vi "STREAM_START.vi"(2 "error in (no error)":errorcluster, 3 "VISA resource Input":refnum<visa-resource-name>) -> (0 "error out":errorcluster, 1 "VISA resource name out":refnum<visa-resource-name>)   [LabVIEW 2011]
panel:
  out "Sent":u8[](array[numeric])
  out "return count":u32
  out "Read  Stream_Start command":u8[](array[numeric])
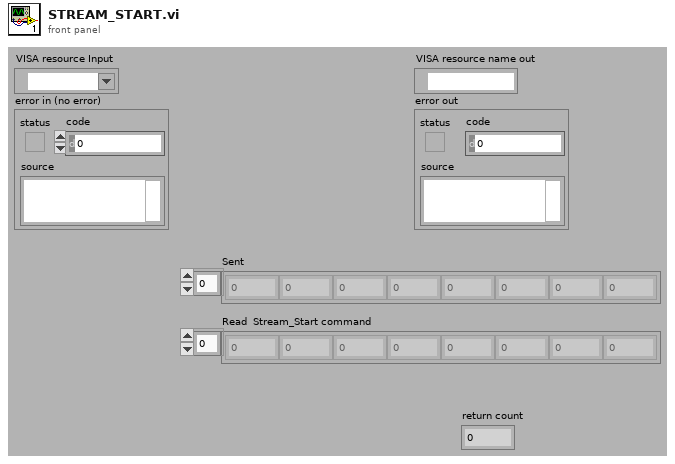
[diagram p1: front panel]
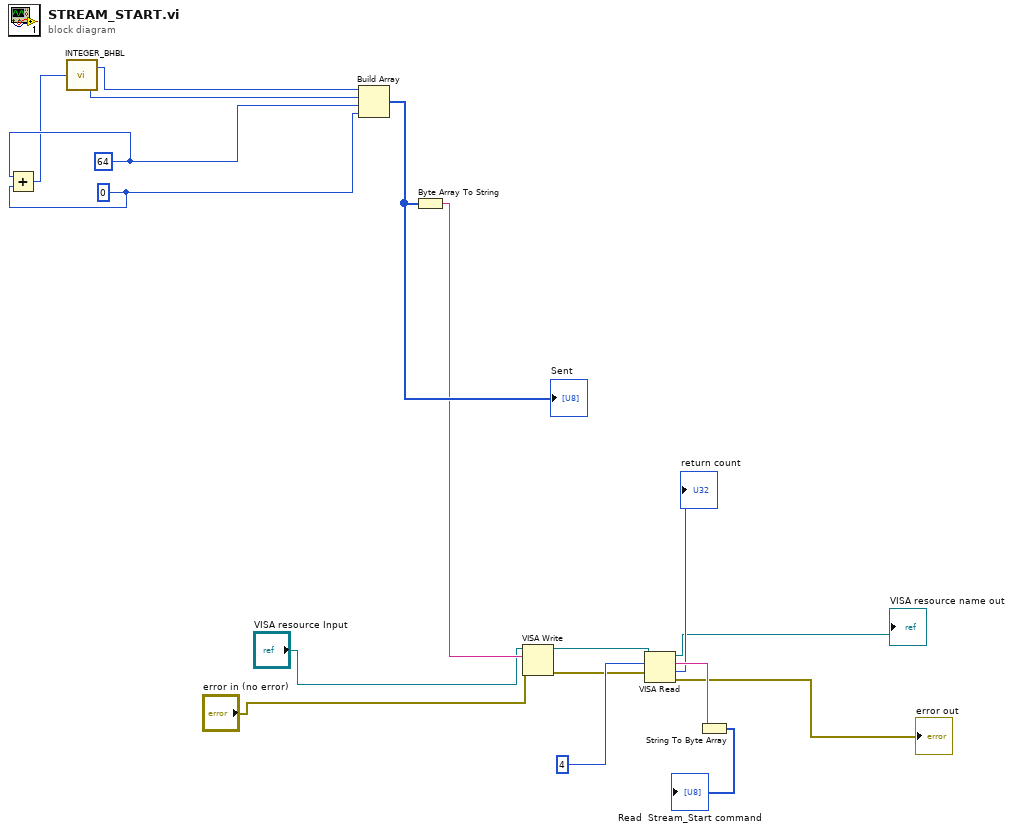
[diagram p0: block diagram]
diagram:
  w5 = i8 0 ("element")
  w4 = i8 64 ("element")
  n1 = Add(x=w4, y=w5) -> (x+y=w3:i8)
  n2 = call "INTEGER_BHBL.vi"("int16"=w3) -> ("Lvalue"=w1:u8, "HValue"=w2:u8)
  n3 = Build Array(w2, w1, w4, w5) -> (w11:u8[])
  "Sent" <- w11
  n4 = Byte Array To String(unsigned byte array=w11) -> (string=w10:string)
  n5 = VISA Write(VISA resource name="VISA resource Input", write buffer=w10, error in (no error)="error in (no error)") -> (VISA resource name out=w13:refnum<visa-resource-name>, error out=w14:errorcluster)  [unwired: 1 out]
  n6 = VISA Read(VISA resource name=w13, byte count=u32 4, error in (no error)=w14) -> (VISA resource name out=→"VISA resource name out":refnum<visa-resource-name>, read buffer=w16:string, return count=→"return count":u32, error out=→"error out":errorcluster)
  n7 = String To Byte Array(string=w16) -> (unsigned byte array=→"Read  Stream_Start command":u8[])
